vi "Store Parameter Value.vi"(8 "PicamParameter":T1=67436581 items=["ExposureTime"=33685527, "ShutterTimingMode"=50593816, "ShutterOpeningDelay"=33685550, "ShutterClosingDelay"=33685529, "ShutterDelayResolution"=50462767, "InternalShutterType"=17039499, "InternalShutterStatus"=17039513, "ExternalShutterType"=17039512, "ExternalShutterStatus"=17039514, "ActiveShutter"=50593947, "InactiveShutterTimingModeResult"=17039516, "GatingMode"=50593885, "RepetitiveGate"=84344926, "SequentialStartingGate"=84344927, "SequentialEndingGate"=84344928, "SequentialGateStepCount"=33947745, "SequentialGateStepIterations"=33947746, "DifStartingGate"=84344934, "DifEndingGate"=84344935, "EnableIntensifier"=50528342, "IntensifierStatus"=17039447, "IntensifierGain"=33620056, "EMIccdGainControlMode"=50593915, "EMIccdGain"=33620092, "PhosphorDecayDelay"=33685593, "PhosphorDecayDelayResolution"=50462810, "BracketGating"=50528356, "IntensifierOptions"=17039461, "EnableModulation"=50528367, "ModulationDuration"=33685622, "ModulationFrequency"=33685616, "RepetitiveModulationPhase"=33685617, "SequentialStartingModulationPhase"=33685618, "SequentialEndingModulationPhase"=33685619, "CustomModulationSequence"=134742135, "PhotocathodeSensitivity"=17039467, "GatingSpeed"=17039468, "PhosphorType"=17039469, "IntensifierDiameter"=16908398, "AdcSpeed"=50462753, "AdcBitDepth"=50397218, "AdcAnalogGain"=50593827, "AdcQuality"=50593828, "AdcEMGain"=33620021, "CorrectPixelBias"=50528362, "TriggerSource"=50593871, "TriggerResponse"=50593822, "TriggerDetermination"=50593823, "TriggerFrequency"=33685584, "TriggerTermination"=50593873, "TriggerCoupling"=50593874, "TriggerThreshold"=33685587, "TriggerDelay"=33685668, "OutputSignal"=50593824, "InvertOutputSignal"=50528308, "OutputSignal2"=50593942, "InvertOutputSignal2"=50528407, "EnableAuxOutput"=50528417, "AuxOutput"=84344923, "EnableSyncMaster"=50528340, "SyncMaster2Delay"=33685589, "EnableModulationOutputSignal"=50528372, "ModulationOutputSignalFrequency"=33685621, "ModulationOutputSignalAmplitude"=33685624, "AnticipateTrigger"=50528387, "DelayFromPreTrigger"=33685636, "ReadoutControlMode"=50593818, "ReadoutTimeCalculation"=16908315, "ReadoutPortCount"=50397212, "ReadoutOrientation"=17039414, "KineticsWindowHeight"=33620024, "SeNsRWindowHeight"=33620131, "VerticalShiftRate"=50462733, "Accumulations"=33947740, "EnableNondestructiveReadout"=50528384, "NondestructiveReadoutPeriod"=33685633, "Rois"=67436581, "NormalizeOrientation"=50528295, "DisableDataFormatting"=50528311, "ReadoutCount"=33947688, "ExactReadoutCountMaximum"=17170509, "PhotonDetectionMode"=50593917, "PhotonDetectionThreshold"=33685630, "PixelFormat"=50593833, "FrameSize"=16842794, "FrameStride"=16842795, "FramesPerReadout"=16842796, "ReadoutStride"=16842797, "PixelBitDepth"=16842800, "ReadoutRateCalculation"=16908338, "OnlineReadoutRateCalculation"=16908387, "FrameRateCalculation"=16908339, "Orientation"=17039398, "TimeStamps"=50593860, "TimeStampResolution"=50724933, "TimeStampBitDepth"=50397254, "TrackFrames"=50528327, "FrameTrackingBitDepth"=50397256, "GateTracking"=50593896, "GateTrackingBitDepth"=50397289, "ModulationTracking"=50593913, "ModulationTrackingBitDepth"=50397306, "SensorType"=17039417, "CcdCharacteristics"=17039418, "SensorActiveWidth"=16842811, "SensorActiveHeight"=16842812, "SensorActiveExtendedHeight"=16842911, "SensorActiveLeftMargin"=16842813, "SensorActiveTopMargin"=16842814, "SensorActiveRightMargin"=16842815, "SensorActiveBottomMargin"=16842816, "SensorMaskedHeight"=16842817, "SensorMaskedTopMargin"=16842818, "SensorMaskedBottomMargin"=16842819, "SensorSecondaryMaskedHeight"=16842801, "SensorSecondaryActiveHeight"=16842826, "PixelWidth"=16908297, "PixelHeight"=16908298, "PixelGapWidth"=16908299, "PixelGapHeight"=16908300, "ApplicableStarDefectMapID"=16842918, "ActiveWidth"=33619969, "ActiveHeight"=33619970, "ActiveExtendedHeight"=33620128, "ActiveLeftMargin"=33619971, "ActiveTopMargin"=33619972, "ActiveRightMargin"=33619973, "ActiveBottomMargin"=33619974, "MaskedHeight"=33619975, "MaskedTopMargin"=33619976, "MaskedBottomMargin"=33620041, "SecondaryMaskedHeight"=33620043, "SecondaryActiveHeight"=33620044, "CleanSectionFinalHeight"=33619985, "CleanSectionFinalHeightCount"=33619986, "CleanSerialRegister"=50528275, "CleanCycleCount"=33619988, "CleanCycleHeight"=33619989, "CleanBeforeExposure"=50528334, "CleanUntilTrigger"=50528278, "StopCleaningOnPreTrigger"=50528386, "SensorTemperatureSetPoint"=33685518, "SensorTemperatureReading"=16908303, "SensorTemperatureStatus"=17039376, "DisableCoolingFan"=50528285, "CoolingFanStatus"=17039522, "EnableSensorWindowHeater"=50528383, "VacuumStatus"=17039525, "CenterWavelengthSetPoint"=33685644, "CenterWavelengthReading"=16908429, "CenterWavelengthStatus"=17039509, "GratingType"=17039502, "GratingCoating"=17039503, "GratingGrooveDensity"=16908432, "GratingBlazingWavelength"=16908433, "FocalLength"=16908434, "InclusionAngle"=16908435, "SensorAngle"=16908436, "LightSource"=50593925, "LightSourceStatus"=17039494, "Age"=16908423, "LifeExpectancy"=16908424, "LaserOutputMode"=50593929, "LaserPower"=33685642, "LaserStatus"=17039517, "InputTriggerStatus"=17039518], 10 "Variant":variant, 11 "Data Cluster in":T2) -> (3 "Data Cluster out":T2)   [LabVIEW 2020, in "Camera.lvlib"]
uses:
  Camera.lvlib
  Module Data--cluster.ctl
  Camera-LVClass/Picam_class/Picam.lvclass
  picam32_LabView_SDK/PICam_lib/types/PicamGatingMode.ctl
  picam32_LabView_SDK/PICam_lib/types/PicamPulse.ctl
  picam32_LabView_SDK/PICam_lib/Ctrls/PicamAdcAnalogGain.ctl
  picam32_LabView_SDK/PICam_lib/Ctrls/PicamAdcQuality.ctl
  picam32_LabView_SDK/PICam_lib/types/PicamIntensifierStatus.ctl
  picam32_LabView_SDK/PICam_lib/types/PicamEMIccdGainControlMode.ctl
  picam32_LabView_SDK/PICam_lib/types/PicamGatingSpeed.ctl
  picam32_LabView_SDK/PICam_lib/types/PicamSensorTemperatureStatus.ctl
  ROI--cluster.ctl
  picam32_LabView_SDK/PICam_lib/types/PicamParameter.ctl
  picam32_LabView_SDK/PICam_lib/PICam.lvlib
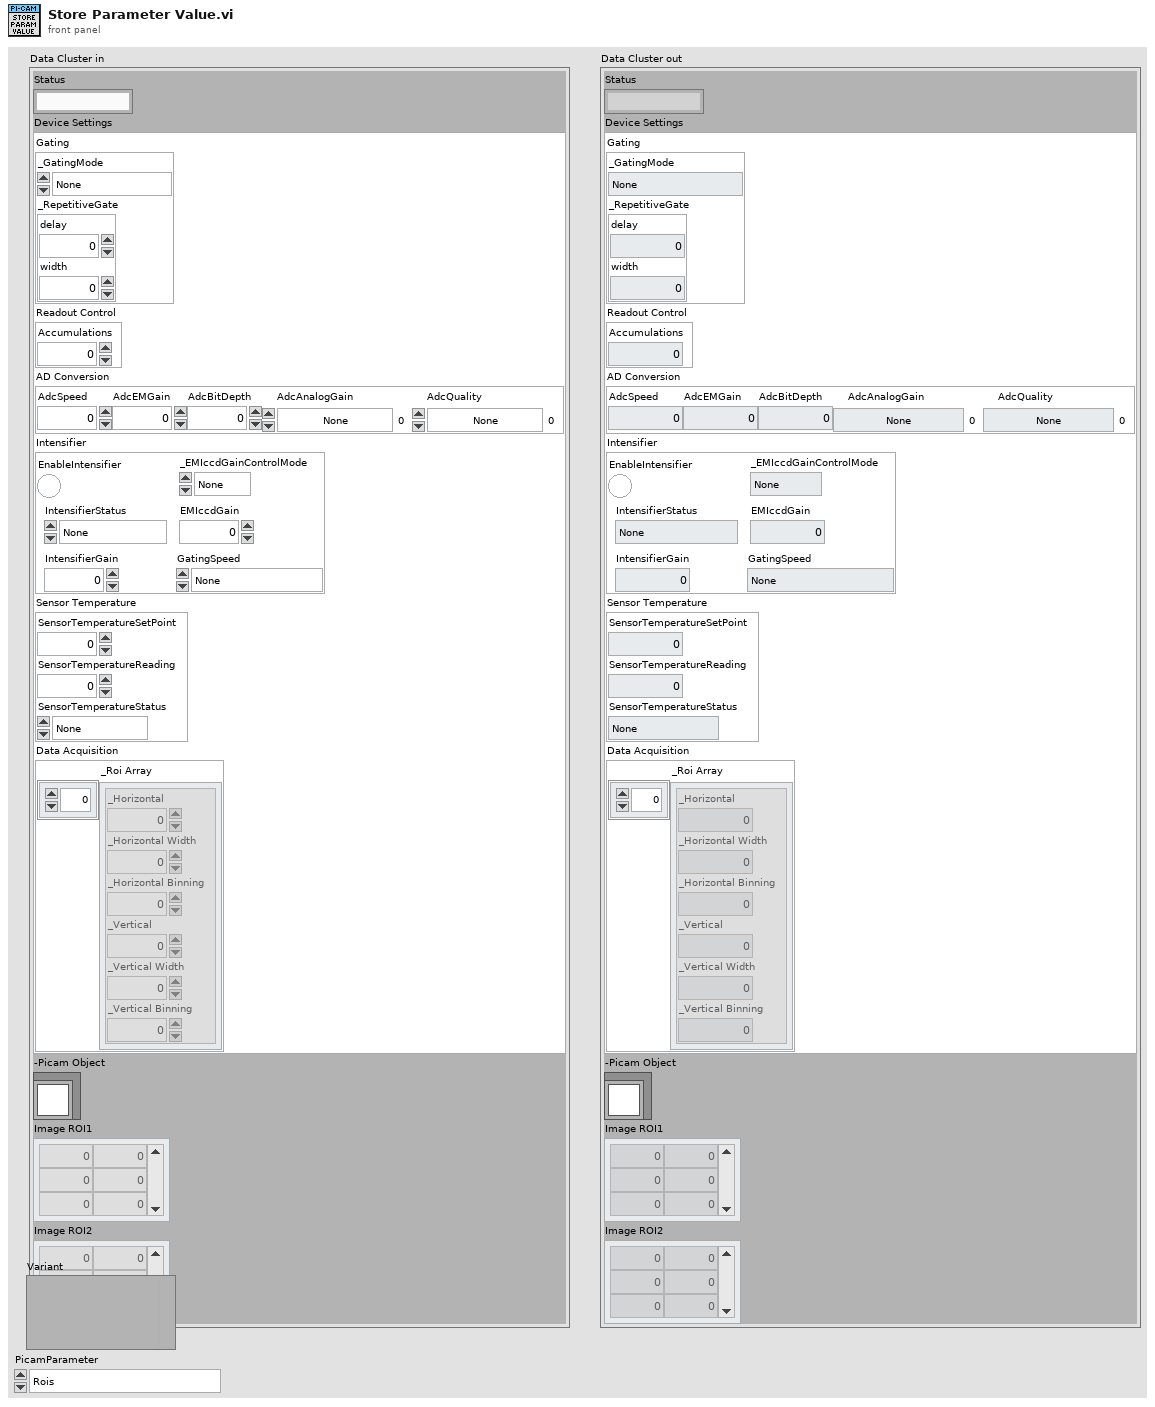
[diagram p1: front panel]
types:
  T1 = typedef "PICam.lvlib/PicamParameter.ctl" = i32
  T2 = typedef "Camera.lvlib/Module Data--cluster.ctl" = cluster{"Status":string, "Device Settings":cluster{"Gating":cluster{"_GatingMode":T3, "_RepetitiveGate":T4}, "Readout Control":cluster{"Accumulations":i64}, "AD Conversion":cluster{"AdcSpeed":dbl, "AdcEMGain":i32, "AdcBitDepth":i32, "AdcAnalogGain":T5, "AdcQuality":T6}, "Intensifier":cluster{"EnableIntensifier":bool, "IntensifierStatus":T7, "IntensifierGain":i32, "_EMIccdGainControlMode":T8, "EMIccdGain":i32, "GatingSpeed":T9}, "Sensor Temperature":cluster{"SensorTemperatureSetPoint":dbl, "SensorTemperatureReading":dbl, "SensorTemperatureStatus":T10}, "Data Acquisition":cluster{"_Roi Array":T11[]}}, "-Picam Object":refnum<class "Picam.lvclass">, "Image ROI1":u16[][], "Image ROI2":u16[][]}
  T3 = typedef "PICam.lvlib/PicamGatingMode.ctl" = enum16{"None", "Repetitive", "Sequential", "Custom", "Disabled"}
  T4 = typedef "PICam.lvlib/PicamPulse.ctl" = cluster{"delay":dbl, "width":dbl}
  T5 = typedef "PICam.lvlib/PicamAdcAnalogGain.ctl" = enum16{"None", "Low", "Medium", "High"}
  T6 = typedef "PICam.lvlib/PicamAdcQuality.ctl" = enum16{"None", "LowNoise", "HighCapacity", "ElectronMultiplied", "HighSpeed"}
  T7 = typedef "PICam.lvlib/PicamIntensifierStatus.ctl" = enum16{"None", "PoweredOff", "PoweredOn"}
  T8 = typedef "PICam.lvlib/PicamEMIccdGainControlMode.ctl" = enum16{"None", "Optimal", "Manual"}
  T9 = typedef "PICam.lvlib/PicamGatingSpeed.ctl" = enum16{"None", "Fast", "Slow"}
  T10 = typedef "PICam.lvlib/PicamSensorTemperatureStatus.ctl" = enum16{"None", "Unlocked", "Locked", "Faulted"}
  T11 = typedef "Camera.lvlib/ROI--cluster.ctl" = cluster{"_Horizontal":i32, "_Horizontal Width":i32, "_Horizontal Binning":i32, "_Vertical":i32, "_Vertical Width":i32, "_Vertical Binning":i32}
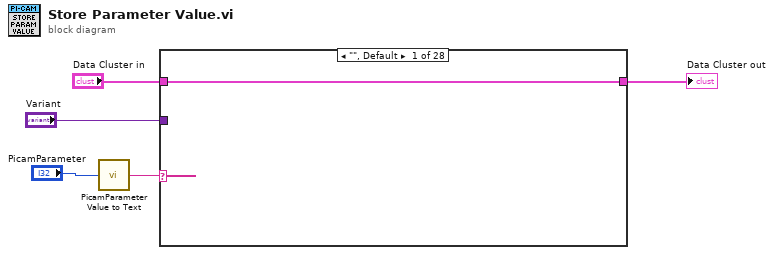
[diagram p0: block diagram]
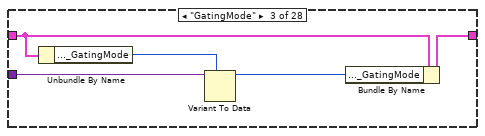
[diagram p3: hidden frame]
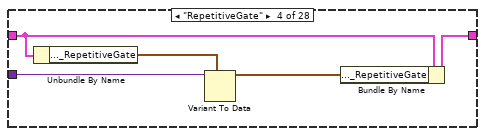
[diagram p4: hidden frame]
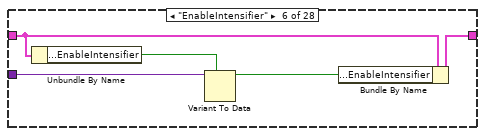
[diagram p6: hidden frame]
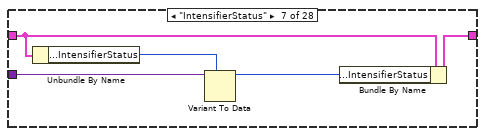
[diagram p7: hidden frame]
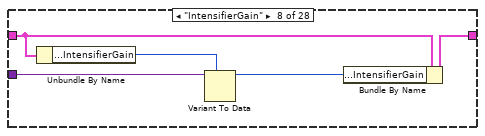
[diagram p8: hidden frame]
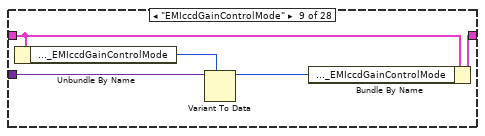
[diagram p9: hidden frame]
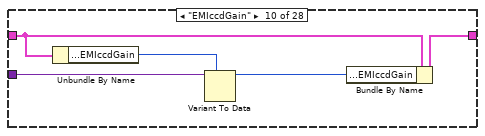
[diagram p10: hidden frame]
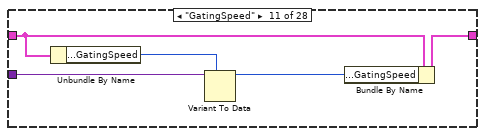
[diagram p11: hidden frame]
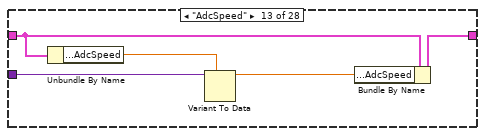
[diagram p13: hidden frame]
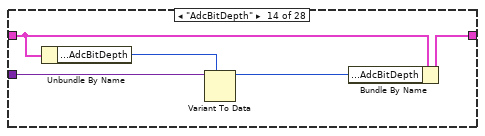
[diagram p14: hidden frame]
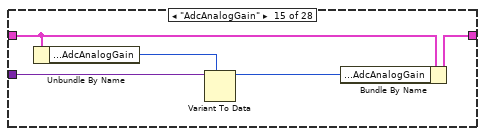
[diagram p15: hidden frame]
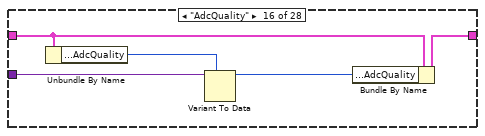
[diagram p16: hidden frame]
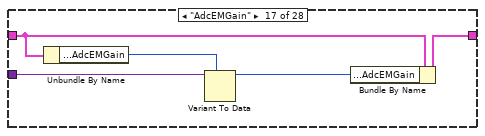
[diagram p17: hidden frame]
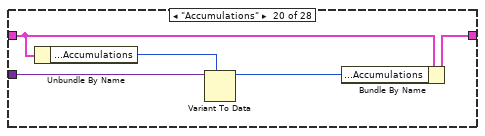
[diagram p20: hidden frame]
diagram:
  n1 = call "PicamParameterValue to Text.vi"("ParameterValue"="PicamParameter") -> ("Parameter Text"=w2:string)
  n2 = case shown="\"\", Default" w2 {
    tunnel: "Variant" -> [_ _ w11 w16 _ w22 w27 w32 w37 w42 w47 _ w53 w58 w63 w68 w73 _ _ w80 _ _ _ _ _ w90 w95 w100]
    tunnel: [w6 w7 w12 w17 w18 w23 w28 w33 w38 w43 w48 w49 w54 w59 w64 w69 w74 w75 w76 w81 w82 w83 w84 w85 w86 w91 w96 w101] -> w5
    tunnel: "Data Cluster in" -> [w6 w7 w10 w15 w18 w21 w26 w31 w36 w41 w46 w49 w52 w57 w62 w67 w72 w75 w76 w79 w82 w83 w84 w85 w86 w89 w94 w99]
    frame "", Default {
    }
    frame "<---Gating--->" {
    }
    frame "GatingMode" {
      n3 = Unbundle By Name(w10) -> ("Device Settings.Gating._GatingMode"=w9:T3)
      n4 = Variant To Data(type=w9, Variant=w11) -> (data=w8:T3)  [unwired: 1 in, 1 out]
      n5 = Bundle By Name(cluster=w10, "Device Settings.Gating._GatingMode"=w8) -> (w12:T2)
    }
    frame "RepetitiveGate" {
      n6 = Unbundle By Name(w15) -> ("Device Settings.Gating._RepetitiveGate"=w14:T4)
      n7 = Variant To Data(type=w14, Variant=w16) -> (data=w13:T4)  [unwired: 1 in, 1 out]
      n8 = Bundle By Name(cluster=w15, "Device Settings.Gating._RepetitiveGate"=w13) -> (w17:T2)
    }
    frame "<---Intensifier--->" {
    }
    frame "EnableIntensifier" {
      n9 = Unbundle By Name(w21) -> ("Device Settings.Intensifier.EnableIntensifier"=w20:bool)
      n10 = Variant To Data(type=w20, Variant=w22) -> (data=w19:bool)  [unwired: 1 in, 1 out]
      n11 = Bundle By Name(cluster=w21, "Device Settings.Intensifier.EnableIntensifier"=w19) -> (w23:T2)
    }
    frame "IntensifierStatus" {
      n12 = Unbundle By Name(w26) -> ("Device Settings.Intensifier.IntensifierStatus"=w25:T7)
      n13 = Variant To Data(type=w25, Variant=w27) -> (data=w24:T7)  [unwired: 1 in, 1 out]
      n14 = Bundle By Name(cluster=w26, "Device Settings.Intensifier.IntensifierStatus"=w24) -> (w28:T2)
    }
    frame "IntensifierGain" {
      n15 = Unbundle By Name(w31) -> ("Device Settings.Intensifier.IntensifierGain"=w30:i32)
      n16 = Variant To Data(type=w30, Variant=w32) -> (data=w29:i32)  [unwired: 1 in, 1 out]
      n17 = Bundle By Name(cluster=w31, "Device Settings.Intensifier.IntensifierGain"=w29) -> (w33:T2)
    }
    frame "EMIccdGainControlMode" {
      n18 = Unbundle By Name(w36) -> ("Device Settings.Intensifier._EMIccdGainControlMode"=w35:T8)
      n19 = Variant To Data(type=w35, Variant=w37) -> (data=w34:T8)  [unwired: 1 in, 1 out]
      n20 = Bundle By Name(cluster=w36, "Device Settings.Intensifier._EMIccdGainControlMode"=w34) -> (w38:T2)
    }
    frame "EMIccdGain" {
      n21 = Unbundle By Name(w41) -> ("Device Settings.Intensifier.EMIccdGain"=w40:i32)
      n22 = Variant To Data(type=w40, Variant=w42) -> (data=w39:i32)  [unwired: 1 in, 1 out]
      n23 = Bundle By Name(cluster=w41, "Device Settings.Intensifier.EMIccdGain"=w39) -> (w43:T2)
    }
    frame "GatingSpeed" {
      n24 = Unbundle By Name(w46) -> ("Device Settings.Intensifier.GatingSpeed"=w45:T9)
      n25 = Variant To Data(type=w45, Variant=w47) -> (data=w44:T9)  [unwired: 1 in, 1 out]
      n26 = Bundle By Name(cluster=w46, "Device Settings.Intensifier.GatingSpeed"=w44) -> (w48:T2)
    }
    frame "<---Analog to Digital Conversion--->" {
    }
    frame "AdcSpeed" {
      n27 = Unbundle By Name(w52) -> ("Device Settings.AD Conversion.AdcSpeed"=w51:dbl)
      n28 = Variant To Data(type=w51, Variant=w53) -> (data=w50:dbl)  [unwired: 1 in, 1 out]
      n29 = Bundle By Name(cluster=w52, "Device Settings.AD Conversion.AdcSpeed"=w50) -> (w54:T2)
    }
    frame "AdcBitDepth" {
      n30 = Unbundle By Name(w57) -> ("Device Settings.AD Conversion.AdcBitDepth"=w56:i32)
      n31 = Variant To Data(type=w56, Variant=w58) -> (data=w55:i32)  [unwired: 1 in, 1 out]
      n32 = Bundle By Name(cluster=w57, "Device Settings.AD Conversion.AdcBitDepth"=w55) -> (w59:T2)
    }
    frame "AdcAnalogGain" {
      n33 = Unbundle By Name(w62) -> ("Device Settings.AD Conversion.AdcAnalogGain"=w61:T5)
      n34 = Variant To Data(type=w61, Variant=w63) -> (data=w60:T5)  [unwired: 1 in, 1 out]
      n35 = Bundle By Name(cluster=w62, "Device Settings.AD Conversion.AdcAnalogGain"=w60) -> (w64:T2)
    }
    frame "AdcQuality" {
      n36 = Unbundle By Name(w67) -> ("Device Settings.AD Conversion.AdcQuality"=w66:T6)
      n37 = Variant To Data(type=w66, Variant=w68) -> (data=w65:T6)  [unwired: 1 in, 1 out]
      n38 = Bundle By Name(cluster=w67, "Device Settings.AD Conversion.AdcQuality"=w65) -> (w69:T2)
    }
    frame "AdcEMGain" {
      n39 = Unbundle By Name(w72) -> ("Device Settings.AD Conversion.AdcEMGain"=w71:i32)
      n40 = Variant To Data(type=w71, Variant=w73) -> (data=w70:i32)  [unwired: 1 in, 1 out]
      n41 = Bundle By Name(cluster=w72, "Device Settings.AD Conversion.AdcEMGain"=w70) -> (w74:T2)
    }
    frame "<---Hardware I/O--->" {
    }
    frame "<---Readout Control--->" {
    }
    frame "Accumulations" {
      n42 = Unbundle By Name(w79) -> ("Device Settings.Readout Control.Accumulations"=w78:i64)
      n43 = Variant To Data(type=w78, Variant=w80) -> (data=w77:i64)  [unwired: 1 in, 1 out]
      n44 = Bundle By Name(cluster=w79, "Device Settings.Readout Control.Accumulations"=w77) -> (w81:T2)
    }
    frame "<---Data Acquisition--->" {
    }
    frame "<---Sensor Information--->" {
    }
    frame "<---Sensor Layout--->" {
    }
    frame "<---Sensor Cleaning--->" {
    }
    frame "<---Sensor Temperature--->" {
    }
    frame "SensorTemperatureSetPoint" {
      n45 = Unbundle By Name(w89) -> ("Device Settings.Sensor Temperature.SensorTemperatureSetPoint"=w88:dbl)
      n46 = Variant To Data(type=w88, Variant=w90) -> (data=w87:dbl)  [unwired: 1 in, 1 out]
      n47 = Bundle By Name(cluster=w89, "Device Settings.Sensor Temperature.SensorTemperatureSetPoint"=w87) -> (w91:T2)
    }
    frame "SensorTemperatureReading" {
      n48 = Unbundle By Name(w94) -> ("Device Settings.Sensor Temperature.SensorTemperatureReading"=w93:dbl)
      n49 = Variant To Data(type=w93, Variant=w95) -> (data=w92:dbl)  [unwired: 1 in, 1 out]
      n50 = Bundle By Name(cluster=w94, "Device Settings.Sensor Temperature.SensorTemperatureReading"=w92) -> (w96:T2)
    }
    frame "SensorTemperatureStatus" {
      n51 = Unbundle By Name(w99) -> ("Device Settings.Sensor Temperature.SensorTemperatureStatus"=w98:T10)
      n52 = Variant To Data(type=w98, Variant=w100) -> (data=w97:T10)  [unwired: 1 in, 1 out]
      n53 = Bundle By Name(cluster=w99, "Device Settings.Sensor Temperature.SensorTemperatureStatus"=w97) -> (w101:T2)
    }
  }
  "Data Cluster out" <- w5
